vi "Flush_FIFOs.vi"() -> (0 "Error Out":u8, 1 "Aborted":bool)   [LabVIEW 2024]
uses:
  <vilib>/rvi/DataTransferAndStorage/Container/XNode/niFpgaContainer.xnode
  <vilib>/rvi/interface/RandomDataEmulation/nirviRandomDataFpgaReadWriteTemplate.vi
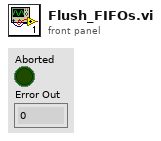
[diagram p1: front panel]
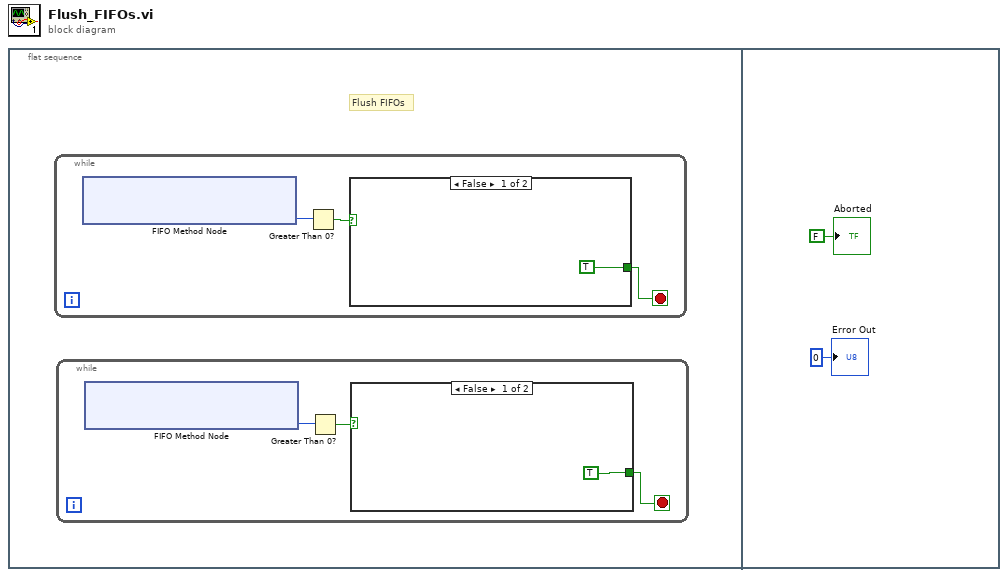
[diagram p0: block diagram]
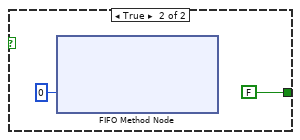
[diagram p2: hidden frame]
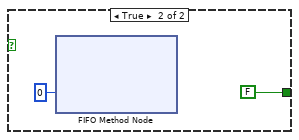
[diagram p3: hidden frame]
diagram:
  n1 = flat-sequence {
    frame #0 {
      # "Flush FIFOs"
      n2 = while {
        stop <- w7 stop-if-true
        n3 = xnode ("FIFO Method Node")() -> ("Number of Elements to Read"=w9:u32)  [unwired: 1 in, 1 out]
        n4 = Greater Than 0?(x=w9) -> (x > 0?=w8:bool)
        n5 = case shown="False" w8 {
          tunnel: [TRUE FALSE] -> w7
          frame False {
          }
          frame True {
            n6 = xnode ("FIFO Method Node")("Timeout"=0) -> ()  [unwired: 1 in, 3 out]
          }
        }
      }
      n7 = while {
        stop <- w1 stop-if-true
        n8 = xnode ("FIFO Method Node")() -> ("Number of Elements to Read"=w3:u32)  [unwired: 1 in, 1 out]
        n9 = Greater Than 0?(x=w3) -> (x > 0?=w2:bool)
        n10 = case shown="False" w2 {
          tunnel: [TRUE FALSE] -> w1
          frame False {
          }
          frame True {
            n11 = xnode ("FIFO Method Node")("Timeout"=0) -> ()  [unwired: 1 in, 3 out]
          }
        }
      }
    }
    frame #1 {
      "Aborted" <- FALSE
      "Error Out" <- u8 0
    }
  }
